vi "Cluster.vi"() -> ()   [LabVIEW 2017]
panel:
  in  "簇":cluster{"数值":dbl, "布尔":bool, "字符串":string}
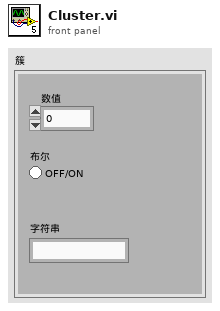
[diagram p1: front panel]
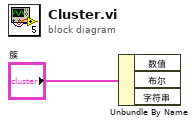
[diagram p0: block diagram]
diagram:
  n1 = Unbundle By Name("簇") -> ()  [unwired: 3 out]
